vi "SPI State Controller Logic.vi"(4 "Frame Complete?":bool, 6 "Enable?":bool, 8 "Sample on trailing edge (Phase)?":bool, 9 "Falling edge leads (Polarity)?":bool, 10 "Start?":bool, 11 "State":T1) -> (0 "Increment?":bool, 2 "Busy?":bool, 3 "State+":T1)   [LabVIEW 2015]
uses:
  SPI States.ctl
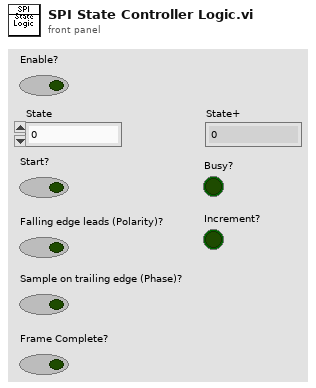
[diagram p1: front panel]
types:
  T1 = typedef "SPI States.ctl" = fxp<+,3,3>
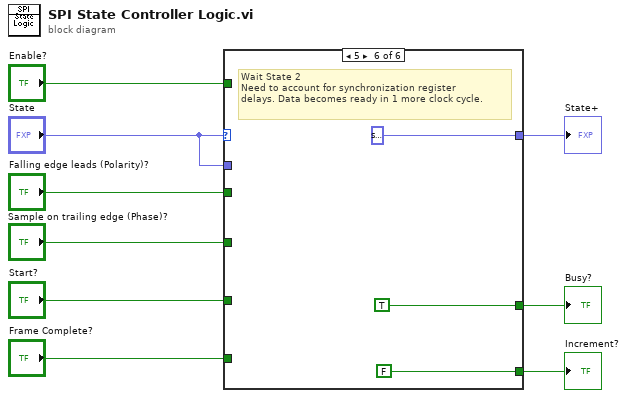
[diagram p0: block diagram]
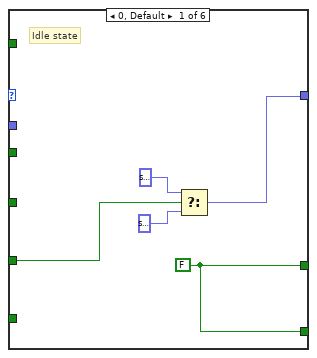
[diagram p2: hidden frame]
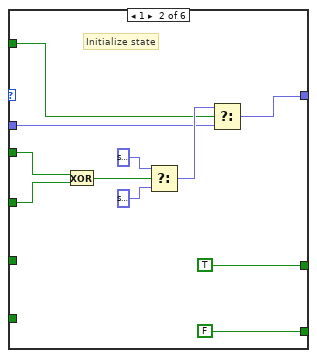
[diagram p3: hidden frame]
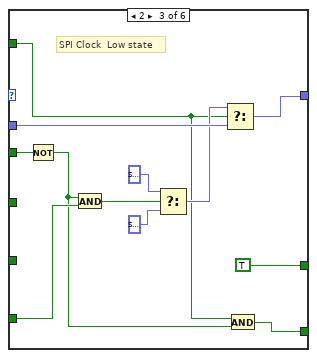
[diagram p4: hidden frame]
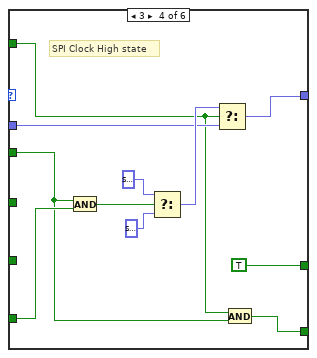
[diagram p5: hidden frame]
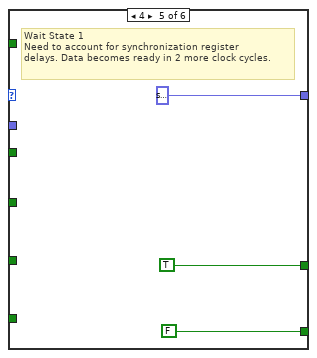
[diagram p6: hidden frame]
diagram:
  n1 = case shown="5" "State" {
    tunnel: "Start?" -> [w14 _ _ _ _ _]
    tunnel: "Falling edge leads (Polarity)?" -> [_ w25 w35 w41 _ _]
    tunnel: [w12 w19 w36 w43 T1 5.0 ("State") T1 0.0 ("State")] -> w7
    tunnel: "Enable?" -> [_ w17 w27 w40 _ _]
    tunnel: "State" -> [_ w18 w37 w44 _ _]
    tunnel: "Frame Complete?" -> [_ _ w34 w48 _ _]
    tunnel: [w10 TRUE TRUE TRUE TRUE TRUE] -> w3
    tunnel: "Sample on trailing edge (Phase)?" -> [_ w24 _ _ _ _]
    tunnel: [w10 FALSE w28 w39 FALSE FALSE] -> w1
    frame 0, Default {
      w10 = FALSE
      # "Idle state"
      n2 = Select(t=T1 1.0, s=w14, f=T1 0.0 ("State")) -> (s? t:f=w12:T1)
    }
    frame 1 {
      # "Initialize state"
      n3 = Exclusive Or(1:w24, 2:w25) -> (0:w23:bool)
      n4 = Select(t=T1 2.0 ("State"), s=w23, f=T1 3.0 ("State")) -> (s? t:f=w20:T1)
      n5 = Select(t=w20, s=w17, f=w18) -> (s? t:f=w19:T1)
    }
    frame 2 {
      # "SPI Clock  Low state"
      n6 = Not(x=w35) -> (.not. x?=w30:bool)
      n7 = And(x=w30, y=w34) -> (x .and. y?=w29:bool)
      n8 = Select(t=T1 4.0 ("State"), s=w29, f=T1 3.0 ("State")) -> (s? t:f=w31:T1)
      n9 = Select(t=w31, s=w27, f=w37) -> (s? t:f=w36:T1)
      n10 = And(x=w27, y=w30) -> (x .and. y?=w28:bool)
    }
    frame 3 {
      # "SPI Clock High state"
      n11 = And(x=w41, y=w48) -> (x .and. y?=w42:bool)
      n12 = Select(t=T1 4.0 ("State"), s=w42, f=T1 2.0 ("State")) -> (s? t:f=w45:T1)
      n13 = Select(t=w45, s=w40, f=w44) -> (s? t:f=w43:T1)
      n14 = And(x=w40, y=w41) -> (x .and. y?=w39:bool)
    }
    frame 4 {
      # "Wait State 1\nNeed to account for synchronization register\ndelays. Data becomes ready in 2 more clock cycles."
    }
    frame 5 {
      # "Wait State 2\nNeed to account for synchronization register\ndelays. Data becomes ready in 1 more clock cycle."
    }
  }
  "State+" <- w7
  "Busy?" <- w3
  "Increment?" <- w1
